vi "Data_Write_2.vi"(0 "Command List":T1, 1 "name":string, 2 "Data":string, 3 "error initialize":errorcluster) -> (7 "Refnum Out During Write":refnum<file>, 9 "error out":errorcluster)   [LabVIEW 2015]
uses:
  Data Write Control.ctl
panel:
  out "cancelled 2":bool
  out "path":path
  out "cancelled":bool
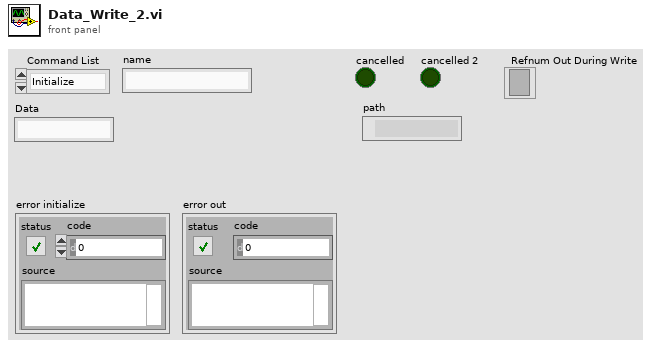
[diagram p1: front panel]
types:
  T1 = typedef "Data Write Control.ctl" = enum16{"Initialize", "Read", "Write", "Close"}
  T2 = enum16{"open", "replace", "create", "open or create", "replace or create", "replace or create with confirmation"}
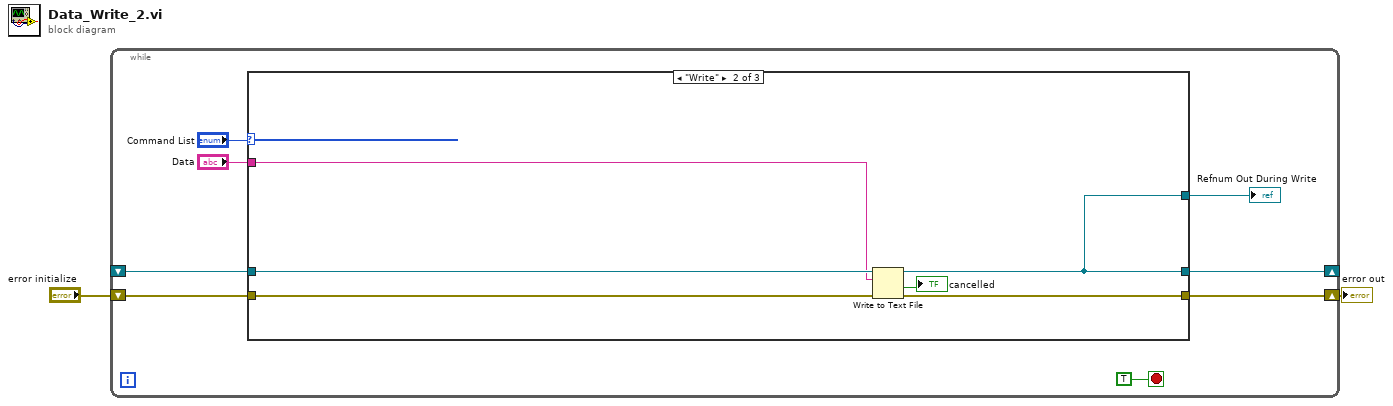
[diagram p0: block diagram]
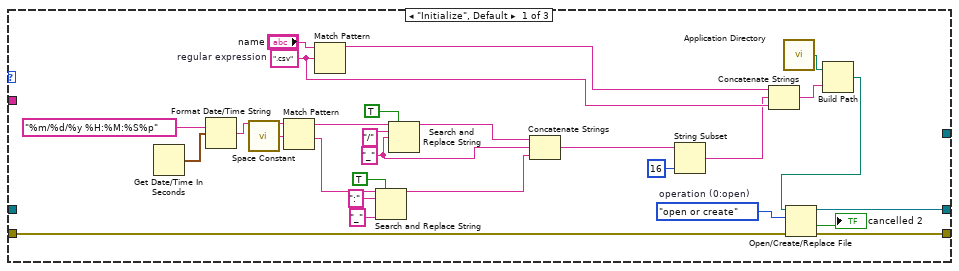
[diagram p2: hidden frame]
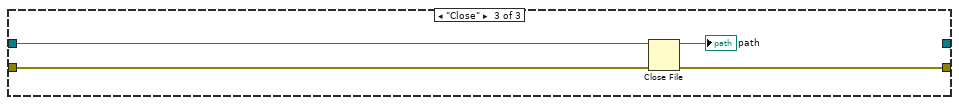
[diagram p3: hidden frame]
diagram:
  n1 = while {
    shift-right: [w7] -> w2
    shift-left: "error initialize" -> [w6]
    shift-right: [w5] -> _
    shift-left: _ -> [w4]
    stop <- TRUE stop-if-true
    n2 = case shown="\"Write\"" "Command List" {
      tunnel: "Data" -> [_ w41 _]
      tunnel: [w38 w44 w48] -> w7
      tunnel: w6 -> [w37 w43 w47]
      tunnel: [w36 w39 _] -> w5
      tunnel: w4 -> [_ w42 w46]
      tunnel: [_ w39 _] -> w3
      frame "Initialize", Default {
        w11 = "_" ("replace string (\"\")")
        w14 = ".csv"  # regular expression
        w33 = T2."open or create"  # operation (0:open)
        n3 = Get Date/Time In Seconds() -> (seconds since 1Jan1904=w31:timestamp)
        n4 = Format Date/Time String(time format string (%c)="%m/%d/%y %H:%M:%S%p", seconds (now)=w31) -> (date/time string=w27:string)  [unwired: 1 in]
        n5 = call <vilib>:"Space Constant.vi"() -> ("String"=w26:string)
        n6 = Match Pattern(string=w27, regular expression=w26) -> (before substring=w25:string, after substring=w23:string)  [unwired: 1 in, 2 out]
        n7 = Match Pattern(string="name", regular expression=w14) -> (before substring=w12:string)  [unwired: 1 in, 3 out]
        n8 = Search and Replace String(replace all?=TRUE ("replace all? (F)"), input string=w23, search string=":", replace string="_" ("replace string (\"\")")) -> (result string=w19:string)  [unwired: 4 in, 3 out]
        n9 = Search and Replace String(replace all?=TRUE ("replace all? (F)"), input string=w25, search string="/", replace string=w11) -> (result string=w20:string)  [unwired: 4 in, 3 out]
        n10 = Concatenate Strings "Concatenate Strings"(w20, w11, w19) -> (w16:string)
        n11 = String Subset(string=w16, length (rest)=16 ("length (rest)")) -> (substring=w13:string)  [unwired: 1 in]
        n12 = Concatenate Strings "Concatenate Strings"(w12, w13, w14) -> (w28:string)
        n13 = call <vilib>:"Application Directory.vi"() -> ("Application Directory"=w32:path)
        n14 = Build Path(base path=w32, name or relative path=w28) -> (appended path=w35:path)
        n15 = Open/Create/Replace File(file path (use dialog)=w35, error in=w37, operation (0:open)=w33) -> (refnum out=w36:refnum<file>, cancelled=→"cancelled 2":bool, error out=w38:errorcluster)  [unwired: 3 in]
      }
      frame "Write" {
        n16 = Write to Text File(file (use dialog)=w42, text=w41, error in=w43) -> (refnum out=w39:refnum<file>, cancelled=→"cancelled":bool, error out=w44:errorcluster)  [unwired: 1 in]
      }
      frame "Close" {
        n17 = Close File(refnum=w46, error in=w47) -> (path=→"path":path, error out=w48:errorcluster)
      }
    }
    "Refnum Out During Write" <- w3
  }
  "error out" <- w2
